vi "Write String.vi"(8 "error in (no error)":errorcluster, 10 "String":string, 11 "NI Digital in":refnum<class "NI Digital to Analog.lvclass">) -> (0 "error out":errorcluster, 3 "NI Digital out":refnum<class "NI Digital to Analog.lvclass">)   [LabVIEW 2018, in "NI Digital to Analog.lvclass"]
doc: "Bus.lvclass:Read String.vi\n\nThis is the template for the Read String VI forthe Bus class.\n\nInstrument Communication Module Version 1.0\nJuly, 2017 Original Code Consulting David Thomson\n www.originalcode.com"
uses:
  NI Digital to Analog/NI Digital to Analog.lvclass
  NI Digital to Analog/NI Digital to Analog.lvclass/NI Digital to Analog.ctl
  <vilib>/DAQmx/write.llb/DAQmx Write (Analog 1D DBL NChan 1Samp).vi
  <vilib>/DAQmx/miscellaneous.llb/DAQmx Fill In Error Info.vi
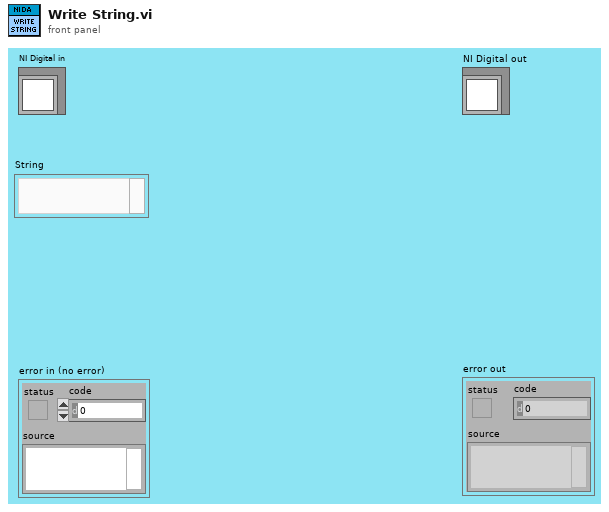
[diagram p1: front panel]
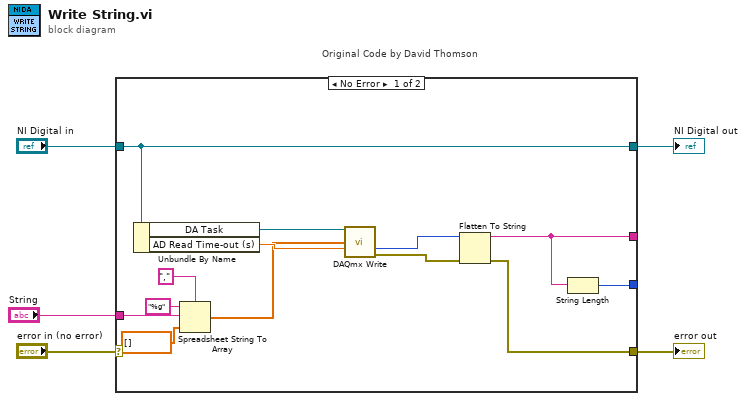
[diagram p0: block diagram]
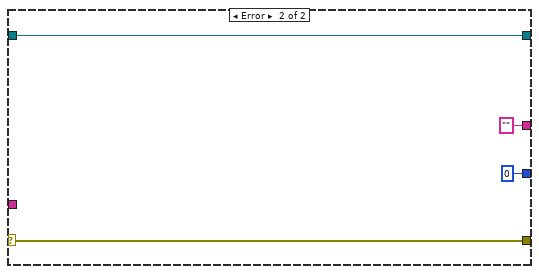
[diagram p2: hidden frame]
diagram:
  n1 = case "Original Code by David Thomson" shown="No Error" "error in (no error)" {
    selector: "error in (no error)" -> [_ w22]
    tunnel: [w13 w22] -> w4
    tunnel: [w17 w21] -> w3
    tunnel: "NI Digital in" -> [w17 w21]
    tunnel: [w12 ""] -> _
    tunnel: [w11 0] -> _
    tunnel: "String" -> [w10 _]
    frame No Error {
      n2 = Unbundle By Name(w17) -> ("DA Task"=w18:refnum<k21>, "AD Read Time-out (s)"=w16:dbl)
      n3 = Spreadsheet String To Array(delimiter (Tab)=",", format string="%g", spreadsheet string=w10, array type (2D Dbl)=dbl[] []) -> (array=w6:dbl[])
      n4 = call-poly <vilib>:"DAQmx Write.vi"("task/channels in"=w18, "data"=w6, "timeout"=w16) -> ("number of samples written per channel"=w15:u32, "error out"=w14:errorcluster)  [unwired: 10 in, 1 out]
      n5 = Flatten To String(anything=w15, error in (no error)=w14) -> (data string=w12:string, error out=w13:errorcluster)  [unwired: 2 in, 1 out]
      n6 = String Length(string=w12) -> (length=w11:i32)
    }
    frame Error {
    }
  }
  "error out" <- w4
  "NI Digital out" <- w3
